vi "pub_simple.vi"   [LabVIEW 2010]
uses:
  socket_type.ctl
  zmq_context.lvclass
  zmq_socket.lvclass
  zeromq.lvlib
panel:
  # "Publishes 5 messages to port 5555\nConnect with client to get messages"
types:
  T1 = typedef "zeromq.lvlib/socket_type.ctl" = enum8{"ZMQ_PAIR", "ZMQ_PUB", "ZMQ_SUB", "ZMQ_REQ", "ZMQ_REP", "ZMQ_DEALER", "ZMQ_ROUTER", "ZMQ_PULL", "ZMQ_PUSH", "ZMQ_XPUB", "ZMQ_XSUB"}
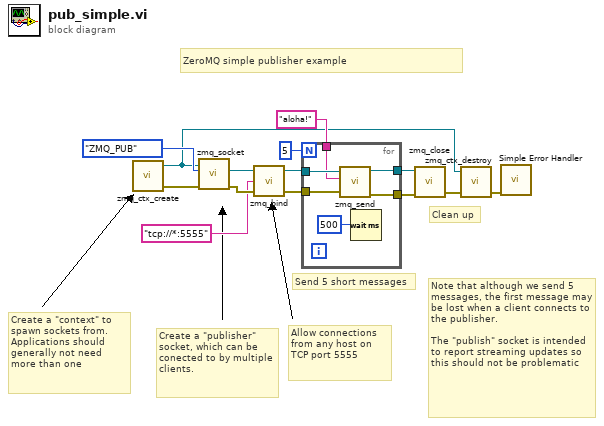
[diagram p0: block diagram]
diagram:
  # "ZeroMQ simple publisher example"
  # "Note that although we send 5 messages, the first message may be lost when a client connects to the publisher.\n\nThe \"publish\" socket is intended to report streaming updates so this should not be problematic"
  # "Clean up"
  # "Send 5 short messages"
  # "Allow connections from any host on TCP port 5555"
  # "Create a \"publisher\" socket, which can be conected to by multiple clients."
  # "Create a \"context\" to spawn sockets from. Applications should generally not need more than one"
  n1 = call "zmq_ctx_create.vi"() -> ("error out"=w12:errorcluster, "context out"=w2:refnum<class "zmq_context.lvclass">)  [unwired: 4 in]
  n2 = call "zmq_socket.vi"("error in"=w12, "socket type"=socket_type."ZMQ_PUB", "context in"=w2) -> ("error out"=w11:errorcluster, "socket out"=w1:refnum<class "zmq_socket.lvclass">)  [unwired: 2 in, 1 out]
  n3 = call "zmq_bind.vi"("error in"=w11, "endpoint"="tcp://*:5555", "socket in"=w1) -> ("error out"=w10:errorcluster, "socket out"=w14:refnum<class "zmq_socket.lvclass">)  [unwired: 1 in]
  n4 = for {
    N: 5 -> [_]
    tunnel: w14 -> [w20]
    tunnel: w10 -> [w19]
    tunnel: [w18] -> w8
    tunnel: "aloha!" ("format string") -> [w17]
    tunnel: [w15] -> w4
    n5 = call "zmq_send.vi"("error in"=w19, "data"=w17, "socket in"=w20) -> ("error out"=w15:errorcluster, "socket out"=w18:refnum<class "zmq_socket.lvclass">)  [unwired: 4 in]
    n6 = Wait (ms)(milliseconds to wait=u32 500) -> ()  [unwired: 1 out]
  }
  n7 = call "zmq_close.vi"("error in"=w4, "socket"=w8) -> ("error out"=w5:errorcluster)  [unwired: 3 in]
  n8 = call "zmq_ctx_destroy.vi"("error in"=w5, "context in"=w2) -> ("error out"=w6:errorcluster)  [unwired: 3 in]
  n9 = call <vilib>:"Simple Error Handler.vi"("error in (no error)"=w6) -> ()  [unwired: 4 in, 5 out]
